vi "删除行.vi"(11 "列表":refnum<vi>) -> ()   [LabVIEW 2020]
panel:
  out "选中行":i32
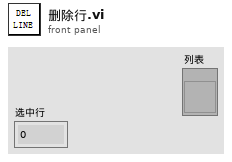
[diagram p1: front panel]
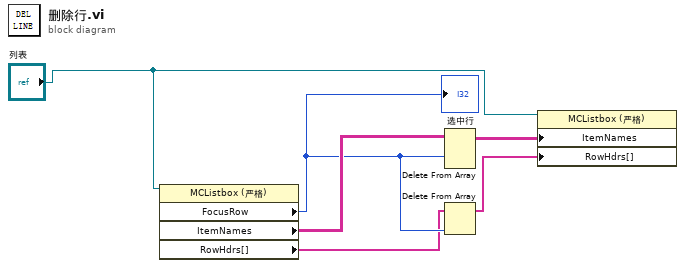
[diagram p0: block diagram]
diagram:
  n1 = property class="MCListbox (严格)"(reference="列表") -> ("FocusRow"=w4:i32, "ItemNames"=w6:string[][], "RowHdrs[]"=w3:string[])  [unwired: 1 in, 2 out]
  "选中行" <- w4
  n2 = Delete From Array(array=w6, index (row)=w4) -> (array with subset deleted=w5:string[][])  [unwired: 2 in, 1 out]
  n3 = Delete From Array(array=w3, index=w4) -> (array with subset deleted=w2:string[])  [unwired: 1 in, 1 out]
  n4 = property class="MCListbox (严格)"(reference="列表", "ItemNames"=w5, "RowHdrs[]"=w2) -> ()  [unwired: 1 in, 2 out]
